vi "GTH-V2.DAC.vi"(5 "ParaList":dbl[](array[numeric])=[4.96841, -0.025143, 0.0], 6 "FileName":string, 7 "CMD":T1(ring), 8 "Error In":errorcluster, 9 "AMP":u8=1 min=1 max=100 step=1, 10 "FREQ":u32=1 min=1 max=65000 step=1, 11 "VISA_USB":refnum<visa-resource-name>) -> (0 "Error Out":errorcluster, 2 "Send CMD":string, 3 "OK?":bool)   [LabVIEW 2012, in "Lib_UEL.ATE.lvlib" / "STM32-CoreBD.lvlib"]
uses:
  STM32-CoreBD.lvlib
  <vilib>/regexp/Match Regular Expression.xnode
panel:
  # "Version History\nV1.0.0 GTH-V2,初始版本. ~ LG,2015-8-14\n- 根据校正参数, 自动根据频率来调值输出幅度.\n- 幅度标准为: 1k@5Vpp,AMP100\n- ON_Chip_Pinknoise, 输出为固定： 450mVrms。\n- 文件输出, wav单声道16bit, 放到根目录,引用方式: /文件名.wav, 不需要双引号. SD卡, 需要使用默认方式格式化.\n- 增加方波输出功能, 支持频率:1~10000Hz \n- 正弦波输出频率为:20~95000Hz"
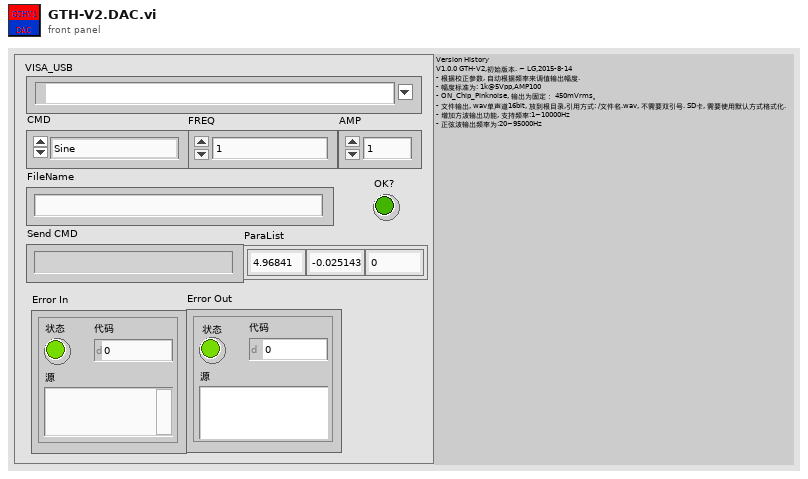
[diagram p1: front panel]
types:
  T1 = enum16{"Sine", "File", "ON_Chip_Pinknoise", "Close Output", "Square"}
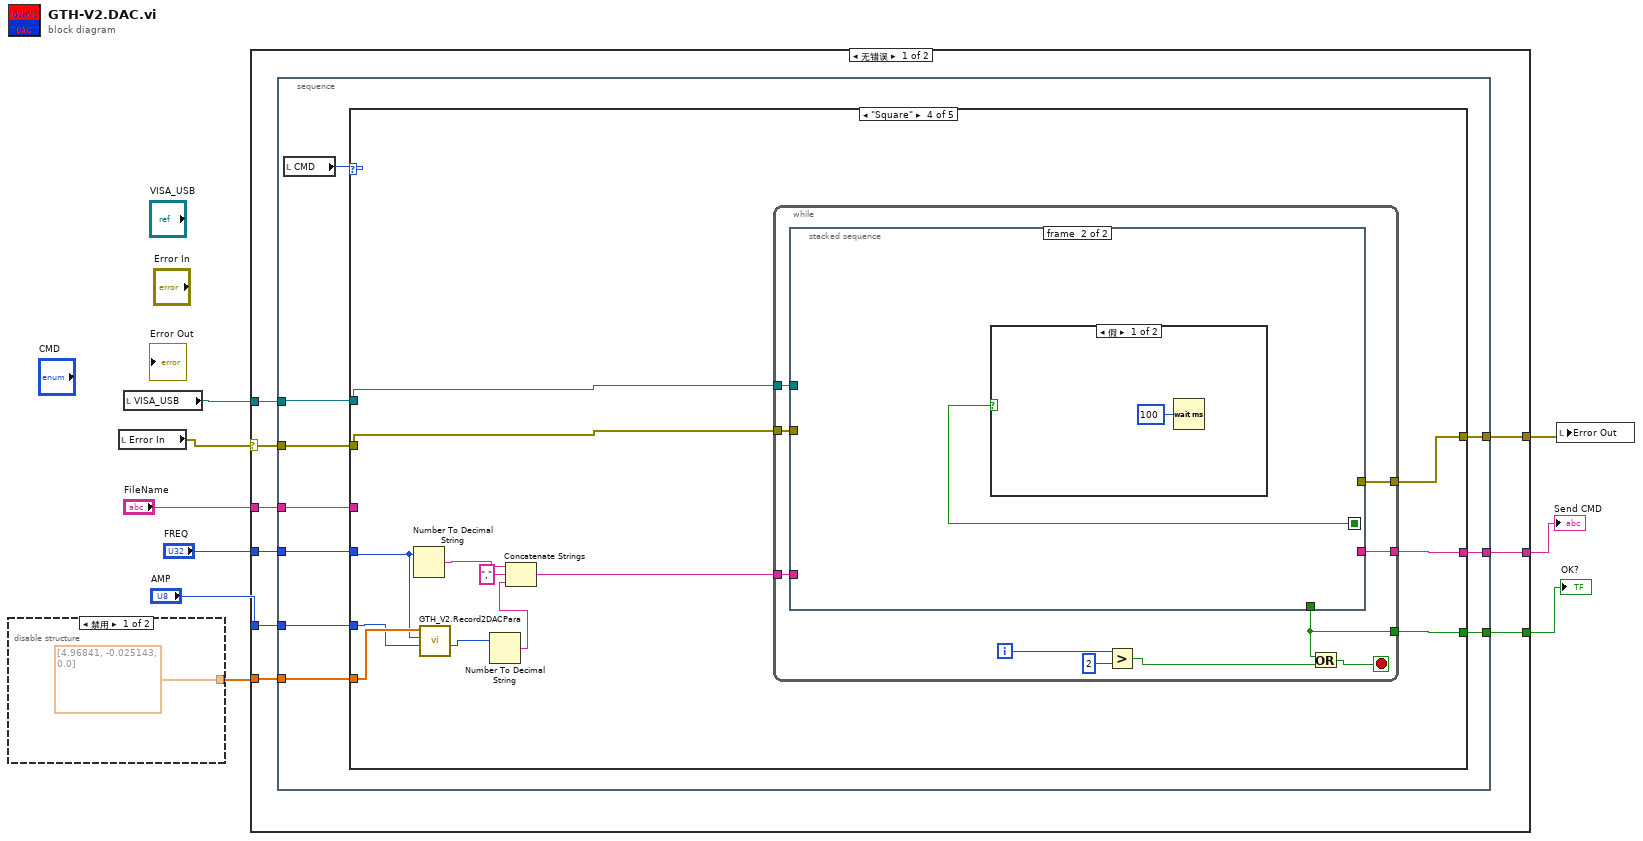
[diagram p0: block diagram]
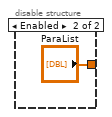
[diagram p2: hidden frame]
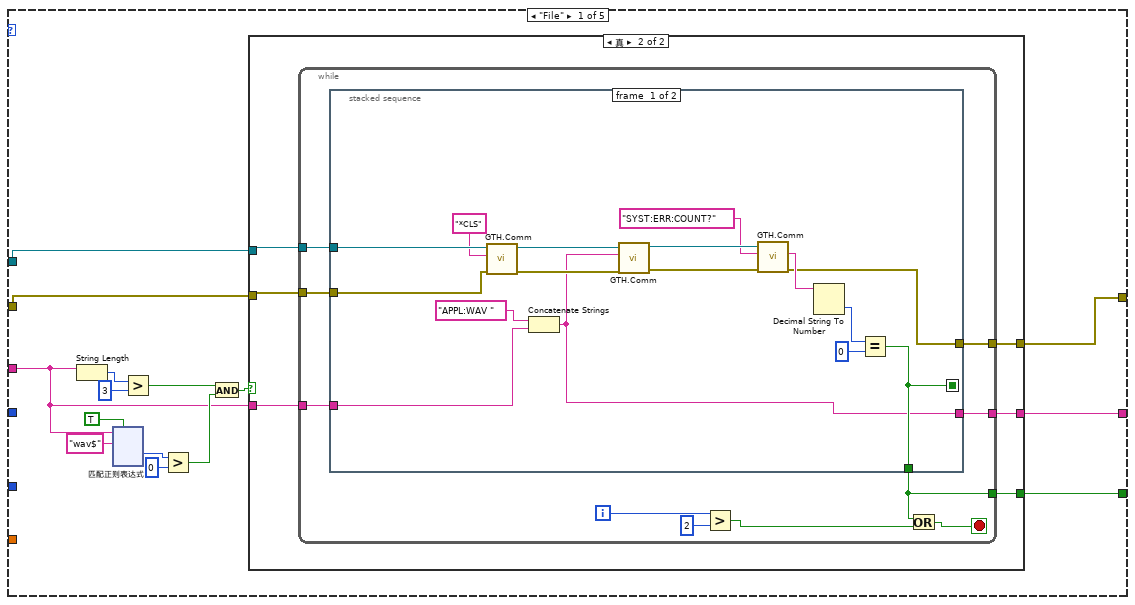
[diagram p3: hidden frame]
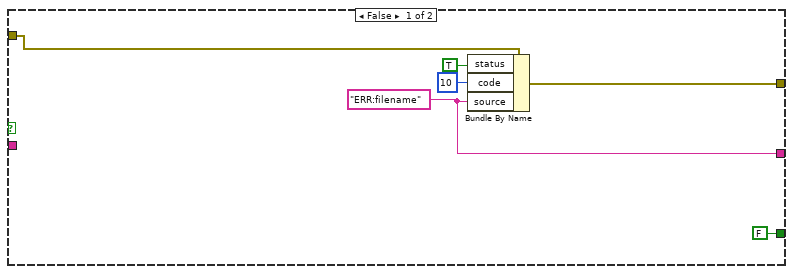
[diagram p4: hidden frame]
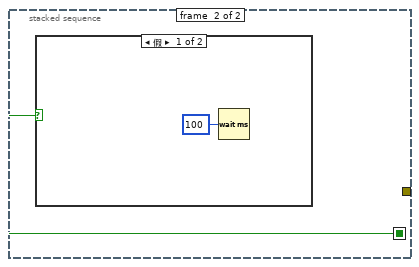
[diagram p5: hidden frame]
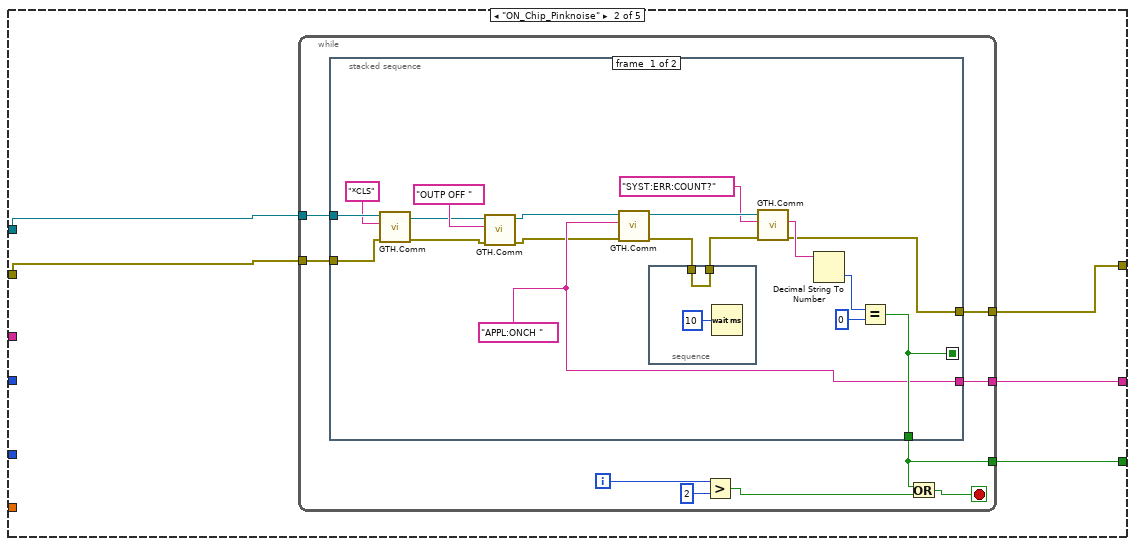
[diagram p7: hidden frame]
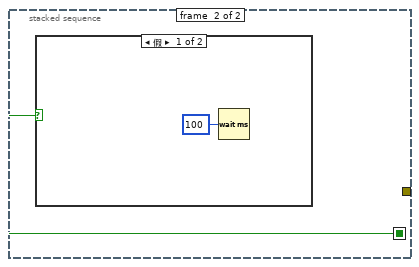
[diagram p8: hidden frame]
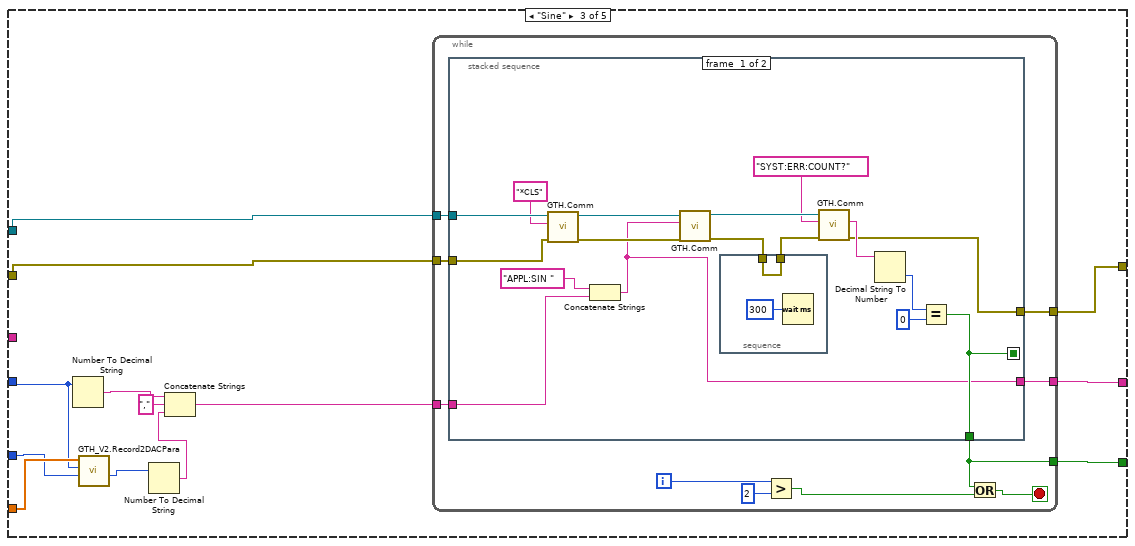
[diagram p10: hidden frame]
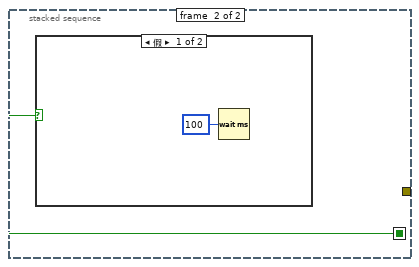
[diagram p11: hidden frame]
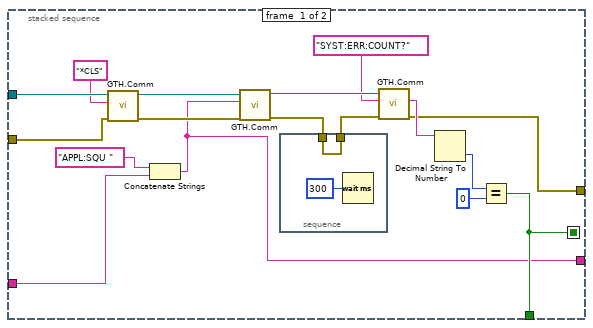
[diagram p13: hidden frame]
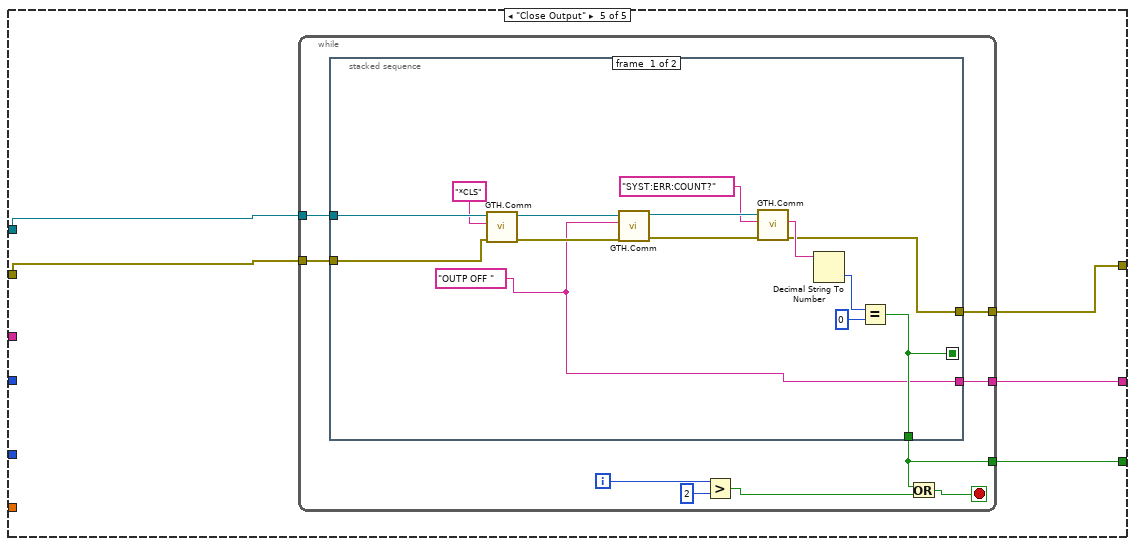
[diagram p15: hidden frame]
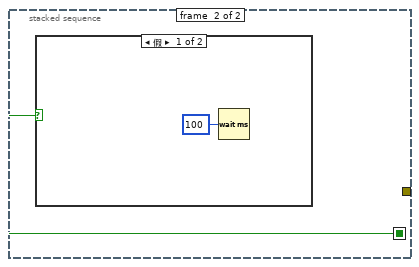
[diagram p16: hidden frame]
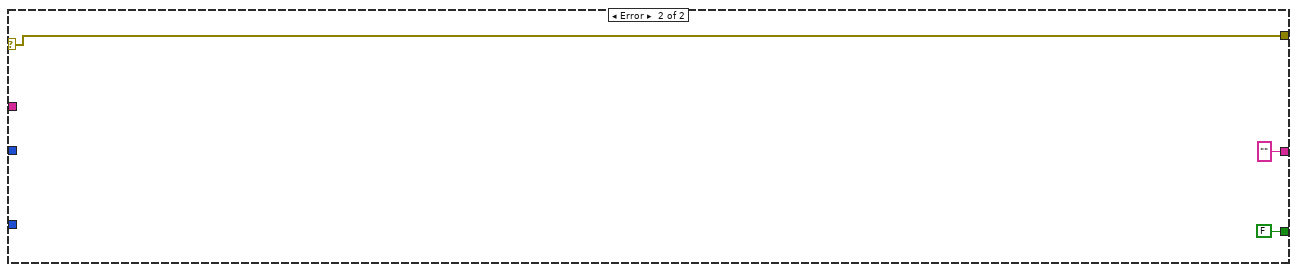
[diagram p18: hidden frame]
diagram:
  n1 = disable-structure shown="禁用" {
    disable-tunnel: [dbl[] [4.96841, -0.025143, 0.0] ("ParaList") "ParaList"] -> w1
    frame Disabled {
    }
    frame Enabled {
    }
  }
  n2 = local read "Error In"() -> (w9:errorcluster)
  n3 = local read "VISA_USB"() -> (w7:refnum<visa-resource-name>)
  n4 = case shown="无错误" w9 {
    selector: w9 -> [w20 w353]
    tunnel: [w19 w353] -> w8
    tunnel: w7 -> [w18 _]
    tunnel: "FileName" -> [w17 _]
    tunnel: [w16 "" ("SCPI CMD")] -> w5
    tunnel: [w15 FALSE] -> w4
    tunnel: "FREQ" -> [w14 _]
    tunnel: "AMP" -> [w13 _]
    tunnel: w1 -> [w12 _]
    frame No Error {
      n5 = stacked-sequence {
        tunnel: w20 -> [w28]
        tunnel: [w27] -> w19
        tunnel: w18 -> [w29]
        tunnel: w17 -> [w26]
        tunnel: [w25] -> w16
        tunnel: [w24] -> w15
        tunnel: w14 -> [w23]
        tunnel: w13 -> [w22]
        tunnel: w12 -> [w21]
        frame #0 {
          n6 = local read "CMD"() -> (w30:T1)
          n7 = case shown="\"Square\"" w30 {
            tunnel: w29 -> [w45 w201 w245 w289 w325]
            tunnel: w28 -> [w44 w200 w244 w288 w324]
            tunnel: [w34 w199 w243 w287 w323] -> w27
            tunnel: w26 -> [w33 _ _ _ _]
            tunnel: [w32 w198 w242 w286 w322] -> w25
            tunnel: [w31 w197 w241 w285 w321] -> w24
            tunnel: w23 -> [_ _ w236 w280 _]
            tunnel: w22 -> [_ _ w235 w279 _]
            tunnel: w21 -> [_ _ w237 w281 _]
            frame "File" {
              n8 = String Length(string=w33) -> (length=w43:i32)
              n9 = xnode "匹配正则表达式"("输入字符串"=w33, "正则表达式"="wav$", "忽略大小写？(F)"=TRUE) -> ("匹配后偏移量"=w39:i32)  [unwired: 3 in, 4 out]
              n10 = Greater?(x=w43, y=3) -> (0:w37:bool)
              n11 = Greater?(x=w39, y=0) -> (0:w36:bool)
              n12 = And(x=w37, y=w36) -> (x .and. y?=w35:bool)
              n13 = case shown="真" w35 {
                tunnel: w45 -> [_ w57]
                tunnel: w44 -> [w51 w56]
                tunnel: [w50 w54] -> w34
                tunnel: w33 -> [_ w55]
                tunnel: [w47 w53] -> w32
                tunnel: [FALSE w52] -> w31
                frame False {
                  w47 = "ERR:filename" ("source")
                  n14 = Bundle By Name(cluster=w51, "status"=TRUE, "code"=10, "source"=w47) -> (w50:errorcluster)
                }
                frame True {
                  n15 = while {
                    tunnel: w57 -> [w67]
                    tunnel: w56 -> [w66]
                    tunnel: w55 -> [w65]
                    tunnel: [w64] -> w54
                    tunnel: [w59] -> w53
                    tunnel: [w58] -> w52
                    i -> [w62]
                    stop <- w63 stop-if-true
                    n16 = stacked-sequence {
                      seq-local: [w69 _] -> [_ w84]
                      tunnel: w67 -> [w83 _]
                      tunnel: w66 -> [w82 _]
                      tunnel: w65 -> [w77 _]
                      tunnel: [w72 _] -> w64
                      tunnel: [w69 _] -> w58
                      tunnel: [w68 _] -> w59
                      frame #0 {
                        n17 = call "GTH.Comm.vi"("Error In"=w82, "SCPI CMD"="*CLS", "USB Port In"=w83) -> ("Error Out"=w79:errorcluster, "USB Port Out"=w80:refnum<visa-resource-name>)  [unwired: 3 in, 4 out]
                        n18 = Concatenate Strings("APPL:WAV " ("SCPI CMD"), w77) -> (w68:string)
                        n19 = call "GTH.Comm.vi"("Error In"=w79, "SCPI CMD"=w68, "USB Port In"=w80) -> ("Error Out"=w75:errorcluster, "USB Port Out"=w76:refnum<visa-resource-name>)  [unwired: 3 in, 4 out]
                        n20 = call "GTH.Comm.vi"("Error In"=w75, "SCPI CMD"="SYST:ERR:COUNT?", "USB Port In"=w76) -> ("Error Out"=w72:errorcluster, "Return"=w73:string)  [unwired: 3 in, 4 out]
                        n21 = Decimal String To Number(string=w73) -> (number=w71:i32)  [unwired: 2 in, 1 out]
                        n22 = Equal?(x=w71, y=0) -> (x = y?=w69:bool)
                      }
                      frame #1 {
                        n23 = case shown="假" w84 {
                          frame False {
                            n24 = Wait (ms)(milliseconds to wait=u32 100 ("等待时间（毫秒）")) -> ()  [unwired: 1 out]
                          }
                          frame True {
                          }
                        }
                      }
                    }
                    n25 = Greater?(x=w62, y=2) -> (0:w60:bool)
                    n26 = Or(x=w58, y=w60) -> (x .or. y?=w63:bool)
                  }
                }
              }
            }
            frame "ON_Chip_Pinknoise" {
              n27 = while {
                tunnel: w201 -> [w210]
                tunnel: w200 -> [w209]
                tunnel: [w208] -> w199
                tunnel: [w203] -> w198
                tunnel: [w202] -> w197
                i -> [w206]
                stop <- w207 stop-if-true
                n28 = stacked-sequence {
                  seq-local: [w219 _] -> [_ w231]
                  tunnel: w210 -> [w228 _]
                  tunnel: w209 -> [w227 _]
                  tunnel: [w222 _] -> w208
                  tunnel: [w219 _] -> w202
                  tunnel: [w218 _] -> w203
                  frame #0 {
                    w218 = "APPL:ONCH " ("SCPI CMD")
                    n29 = call "GTH.Comm.vi"("Error In"=w227, "SCPI CMD"="*CLS", "USB Port In"=w228) -> ("Error Out"=w214:errorcluster, "USB Port Out"=w213:refnum<visa-resource-name>)  [unwired: 3 in, 4 out]
                    n30 = call "GTH.Comm.vi"("Error In"=w214, "SCPI CMD"="OUTP OFF ", "USB Port In"=w213) -> ("Error Out"=w211:errorcluster, "USB Port Out"=w212:refnum<visa-resource-name>)  [unwired: 3 in, 4 out]
                    n31 = call "GTH.Comm.vi"("Error In"=w211, "SCPI CMD"=w218, "USB Port In"=w212) -> ("Error Out"=w217:errorcluster, "USB Port Out"=w225:refnum<visa-resource-name>)  [unwired: 3 in, 4 out]
                    n32 = stacked-sequence {
                      tunnel: [w230] -> w216
                      tunnel: w217 -> [w230]
                      frame #0 {
                        n33 = Wait (ms)(milliseconds to wait=u32 10 ("等待时间（毫秒）")) -> ()  [unwired: 1 out]
                      }
                    }
                    n34 = call "GTH.Comm.vi"("Error In"=w216, "SCPI CMD"="SYST:ERR:COUNT?", "USB Port In"=w225) -> ("Error Out"=w222:errorcluster, "Return"=w223:string)  [unwired: 3 in, 4 out]
                    n35 = Decimal String To Number(string=w223) -> (number=w221:i32)  [unwired: 2 in, 1 out]
                    n36 = Equal?(x=w221, y=0) -> (x = y?=w219:bool)
                  }
                  frame #1 {
                    n37 = case shown="假" w231 {
                      frame False {
                        n38 = Wait (ms)(milliseconds to wait=u32 100 ("等待时间（毫秒）")) -> ()  [unwired: 1 out]
                      }
                      frame True {
                      }
                    }
                  }
                }
                n39 = Greater?(x=w206, y=2) -> (0:w204:bool)
                n40 = Or(x=w202, y=w204) -> (x .or. y?=w207:bool)
              }
            }
            frame "Sine" {
              n41 = Number To Decimal String(number=w236) -> (decimal integer string=w240:string)  [unwired: 1 in]
              n42 = call "GTH_V2.Record2DACPara.vi"("AMP"=w235, "FREQ"=w236, "ParaList"=w237) -> ("AMP OUT"=w234:u8)  [unwired: 8 in]
              n43 = Number To Decimal String(number=w234) -> (decimal integer string=w233:string)  [unwired: 1 in]
              n44 = Concatenate Strings(w240, "," ("字符串"), w233) -> (w238:string)
              n45 = while {
                tunnel: w245 -> [w255]
                tunnel: w244 -> [w254]
                tunnel: [w253] -> w243
                tunnel: [w248] -> w242
                tunnel: [w247] -> w241
                tunnel: w238 -> [w246]
                i -> [w251]
                stop <- w252 stop-if-true
                n46 = stacked-sequence {
                  seq-local: [w260 _] -> [_ w275]
                  tunnel: w255 -> [w272 _]
                  tunnel: w254 -> [w271 _]
                  tunnel: [w263 _] -> w253
                  tunnel: [w260 _] -> w247
                  tunnel: [w259 _] -> w248
                  tunnel: w246 -> [w258 _]
                  frame #0 {
                    n47 = call "GTH.Comm.vi"("Error In"=w271, "SCPI CMD"="*CLS", "USB Port In"=w272) -> ("Error Out"=w268:errorcluster, "USB Port Out"=w269:refnum<visa-resource-name>)  [unwired: 3 in, 4 out]
                    n48 = Concatenate Strings("APPL:SIN " ("SCPI CMD"), w258) -> (w259:string)
                    n49 = call "GTH.Comm.vi"("Error In"=w268, "SCPI CMD"=w259, "USB Port In"=w269) -> ("Error Out"=w256:errorcluster, "USB Port Out"=w266:refnum<visa-resource-name>)  [unwired: 3 in, 4 out]
                    n50 = stacked-sequence {
                      tunnel: [w274] -> w257
                      tunnel: w256 -> [w274]
                      frame #0 {
                        n51 = Wait (ms)(milliseconds to wait=u32 300 ("等待时间（毫秒）")) -> ()  [unwired: 1 out]
                      }
                    }
                    n52 = call "GTH.Comm.vi"("Error In"=w257, "SCPI CMD"="SYST:ERR:COUNT?", "USB Port In"=w266) -> ("Error Out"=w263:errorcluster, "Return"=w264:string)  [unwired: 3 in, 4 out]
                    n53 = Decimal String To Number(string=w264) -> (number=w262:i32)  [unwired: 2 in, 1 out]
                    n54 = Equal?(x=w262, y=0) -> (x = y?=w260:bool)
                  }
                  frame #1 {
                    n55 = case shown="假" w275 {
                      frame False {
                        n56 = Wait (ms)(milliseconds to wait=u32 100 ("等待时间（毫秒）")) -> ()  [unwired: 1 out]
                      }
                      frame True {
                      }
                    }
                  }
                }
                n57 = Greater?(x=w251, y=2) -> (0:w249:bool)
                n58 = Or(x=w247, y=w249) -> (x .or. y?=w252:bool)
              }
            }
            frame "Square" {
              n59 = Number To Decimal String(number=w280) -> (decimal integer string=w284:string)  [unwired: 1 in]
              n60 = call "GTH_V2.Record2DACPara.vi"("AMP"=w279, "FREQ"=w280, "ParaList"=w281) -> ("AMP OUT"=w278:u8)  [unwired: 8 in]
              n61 = Number To Decimal String(number=w278) -> (decimal integer string=w277:string)  [unwired: 1 in]
              n62 = Concatenate Strings(w284, "," ("字符串"), w277) -> (w282:string)
              n63 = while {
                tunnel: w289 -> [w299]
                tunnel: w288 -> [w298]
                tunnel: [w297] -> w287
                tunnel: [w292] -> w286
                tunnel: [w291] -> w285
                tunnel: w282 -> [w290]
                i -> [w295]
                stop <- w296 stop-if-true
                n64 = stacked-sequence {
                  seq-local: [w304 _] -> [_ w319]
                  tunnel: w299 -> [w316 _]
                  tunnel: w298 -> [w315 _]
                  tunnel: [w307 _] -> w297
                  tunnel: [w304 _] -> w291
                  tunnel: [w303 _] -> w292
                  tunnel: w290 -> [w302 _]
                  frame #0 {
                    n65 = call "GTH.Comm.vi"("Error In"=w315, "SCPI CMD"="*CLS", "USB Port In"=w316) -> ("Error Out"=w312:errorcluster, "USB Port Out"=w313:refnum<visa-resource-name>)  [unwired: 3 in, 4 out]
                    n66 = Concatenate Strings("APPL:SQU " ("SCPI CMD"), w302) -> (w303:string)
                    n67 = call "GTH.Comm.vi"("Error In"=w312, "SCPI CMD"=w303, "USB Port In"=w313) -> ("Error Out"=w300:errorcluster, "USB Port Out"=w310:refnum<visa-resource-name>)  [unwired: 3 in, 4 out]
                    n68 = stacked-sequence {
                      tunnel: [w318] -> w301
                      tunnel: w300 -> [w318]
                      frame #0 {
                        n69 = Wait (ms)(milliseconds to wait=u32 300 ("等待时间（毫秒）")) -> ()  [unwired: 1 out]
                      }
                    }
                    n70 = call "GTH.Comm.vi"("Error In"=w301, "SCPI CMD"="SYST:ERR:COUNT?", "USB Port In"=w310) -> ("Error Out"=w307:errorcluster, "Return"=w308:string)  [unwired: 3 in, 4 out]
                    n71 = Decimal String To Number(string=w308) -> (number=w306:i32)  [unwired: 2 in, 1 out]
                    n72 = Equal?(x=w306, y=0) -> (x = y?=w304:bool)
                  }
                  frame #1 {
                    n73 = case shown="假" w319 {
                      frame False {
                        n74 = Wait (ms)(milliseconds to wait=u32 100 ("等待时间（毫秒）")) -> ()  [unwired: 1 out]
                      }
                      frame True {
                      }
                    }
                  }
                }
                n75 = Greater?(x=w295, y=2) -> (0:w293:bool)
                n76 = Or(x=w291, y=w293) -> (x .or. y?=w296:bool)
              }
            }
            frame "Close Output" {
              n77 = while {
                tunnel: w325 -> [w334]
                tunnel: w324 -> [w333]
                tunnel: [w332] -> w323
                tunnel: [w327] -> w322
                tunnel: [w326] -> w321
                i -> [w330]
                stop <- w331 stop-if-true
                n78 = stacked-sequence {
                  seq-local: [w336 _] -> [_ w349]
                  tunnel: w334 -> [w348 _]
                  tunnel: w333 -> [w347 _]
                  tunnel: [w339 _] -> w332
                  tunnel: [w336 _] -> w326
                  tunnel: [w335 _] -> w327
                  frame #0 {
                    w335 = "OUTP OFF " ("SCPI CMD")
                    n79 = call "GTH.Comm.vi"("Error In"=w347, "SCPI CMD"="*CLS", "USB Port In"=w348) -> ("Error Out"=w344:errorcluster, "USB Port Out"=w345:refnum<visa-resource-name>)  [unwired: 3 in, 4 out]
                    n80 = call "GTH.Comm.vi"("Error In"=w344, "SCPI CMD"=w335, "USB Port In"=w345) -> ("Error Out"=w342:errorcluster, "USB Port Out"=w343:refnum<visa-resource-name>)  [unwired: 3 in, 4 out]
                    n81 = call "GTH.Comm.vi"("Error In"=w342, "SCPI CMD"="SYST:ERR:COUNT?", "USB Port In"=w343) -> ("Error Out"=w339:errorcluster, "Return"=w340:string)  [unwired: 3 in, 4 out]
                    n82 = Decimal String To Number(string=w340) -> (number=w338:i32)  [unwired: 2 in, 1 out]
                    n83 = Equal?(x=w338, y=0) -> (x = y?=w336:bool)
                  }
                  frame #1 {
                    n84 = case shown="假" w349 {
                      frame False {
                        n85 = Wait (ms)(milliseconds to wait=u32 100 ("等待时间（毫秒）")) -> ()  [unwired: 1 out]
                      }
                      frame True {
                      }
                    }
                  }
                }
                n86 = Greater?(x=w330, y=2) -> (0:w328:bool)
                n87 = Or(x=w326, y=w328) -> (x .or. y?=w331:bool)
              }
            }
          }
        }
      }
    }
    frame Error {
    }
  }
  "Send CMD" <- w5
  "OK?" <- w4
  n88 = local write "Error Out"(w8) -> ()
